vi "CLD1010 Example.vi"() -> ()   [LabVIEW 2023]
panel:
  in  "Resource Name":refnum<visa-resource-name>="USB0::0x1313::0x804F::M00413716::INSTR"
  out "Temperature High Limit":dbl caption="Setpoint High Limit"
  out "Temperature  Low Limit":dbl caption="Setpoint Low Limit"
  in  "Laser Diode Current Setpoint [A] (0.0)":dbl caption="Laser Diode Current Setpoint (0.0)"
  out "Measured Temperature":dbl caption="Temperature"
  in  "Temperature Setpoint [°C] (25.0)":dbl=25.0 caption="Temperature Setpoint (25.0)"
  # "CLD1010 Example"
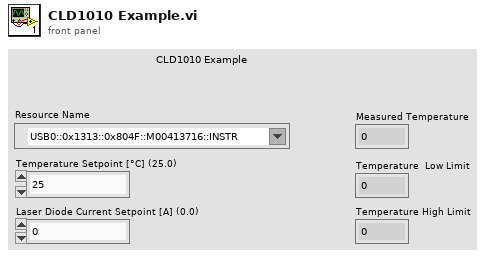
[diagram p1: front panel]
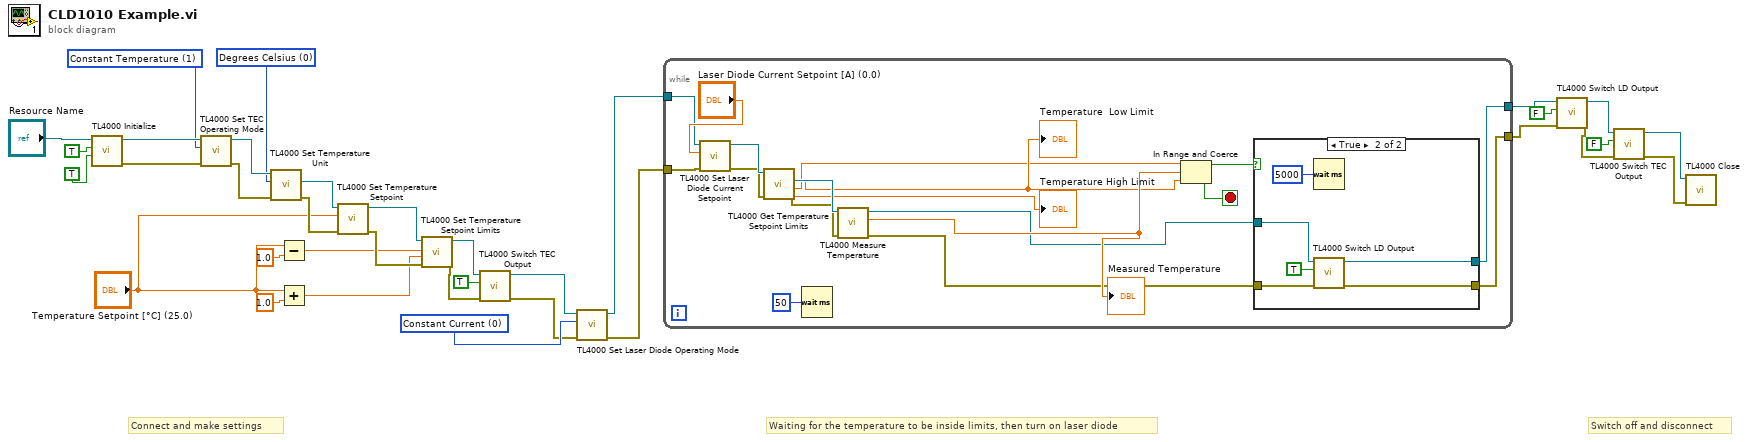
[diagram p0: block diagram]
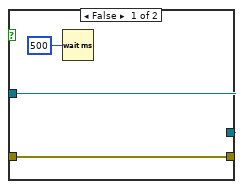
[diagram p2: hidden frame]
diagram:
  w21 = i16 1 items=["Constant Temperature"=1, "Current Source"=0] ("TEC Operating Mode (Constant Temperature)")
  w22 = i16 0 items=["Degrees Celsius", "Kelvin", "Degrees Fahrenheit"] ("Temperature Unit (Degrees Celsius)")
  w27 = i16 0 items=["Constant Current", "Constant Power"] ("Laser Diode Operating Mode (Constant Current)")
  # "Switch off and disconnect"
  # "Waiting for the temperature to be inside limits, then turn on laser diode"
  # "Connect and make settings"
  n1 = call <instrlib>:"TL4000 Initialize.vi"("Reset Device (Reset Device)"=TRUE, "ID Query (Do Query)"=TRUE, "resource name"="Resource Name") -> ("error out"=w1:errorcluster, "instrument handle out"=w31:refnum<visa-resource-name>)  [unwired: 7 in]
  n2 = call <instrlib>:"TL4000 Set TEC Operating Mode.vi"("error in (no error)"=w1, "TEC Operating Mode (Constant Temperature)"=w21, "instrument handle"=w31) -> ("error out"=w24:errorcluster, "instrument handle out"=w26:refnum<visa-resource-name>)  [unwired: 7 in]
  n3 = call <instrlib>:"TL4000 Set Temperature Unit.vi"("error in (no error)"=w24, "Temperature Unit (Degrees Celsius)"=w22, "instrument handle"=w26) -> ("error out"=w23:errorcluster, "instrument handle out"=w25:refnum<visa-resource-name>)  [unwired: 7 in]
  n4 = Subtract(x="Temperature Setpoint [°C] (25.0)", y=1.0) -> (x-y=w2:dbl)
  n5 = Add(x="Temperature Setpoint [°C] (25.0)", y=1.0) -> (x+y=w5:dbl)
  n6 = call <instrlib>:"TL4000 Set Temperature Setpoint.vi"("error in (no error)"=w23, "Temperature Setpoint (25.0)"="Temperature Setpoint [°C] (25.0)", "instrument handle"=w25) -> ("error out"=w8:errorcluster, "instrument handle out"=w10:refnum<visa-resource-name>)  [unwired: 7 in]
  n7 = call "TL4000 Set Temperature Setpoint Limits.vi"("error in (no error)"=w8, "Setpoint High Limit (50.0)"=w5, "Setpoint Low Limit (0.0)"=w2, "instrument handle"=w10) -> ("error out"=w7:errorcluster, "instrument handle out"=w9:refnum<visa-resource-name>)  [unwired: 6 in]
  n8 = call <instrlib>:"TL4000 Switch TEC Output.vi"("error in (no error)"=w7, "TEC Output (Off)"=TRUE, "instrument handle"=w9) -> ("error out"=w19:errorcluster, "instrument handle out"=w20:refnum<visa-resource-name>)  [unwired: 7 in]
  n9 = call <instrlib>:"TL4000 Set Laser Diode Operating Mode.vi"("error in (no error)"=w19, "Laser Diode Operating Mode (Constant Current)"=w27, "instrument handle"=w20) -> ("error out"=w29:errorcluster, "instrument handle out"=w28:refnum<visa-resource-name>)  [unwired: 7 in]
  n10 = while {
    tunnel: w29 -> [w44]
    tunnel: w28 -> [w45]
    tunnel: [w42] -> w15
    tunnel: [w41] -> w14
    stop <- w43 stop-if-true
    n11 = call <instrlib>:"TL4000 Set Laser Diode Current Setpoint.vi"("error in (no error)"=w44, "Laser Diode Current Setpoint (0.0)"="Laser Diode Current Setpoint [A] (0.0)", "instrument handle"=w45) -> ("error out"=w39:errorcluster, "instrument handle out"=w40:refnum<visa-resource-name>)  [unwired: 7 in]
    n12 = call "TL4000 Get Temperature Setpoint Limits.vi"("error in (no error)"=w39, "instrument handle"=w40) -> ("error out"=w37:errorcluster, "Setpoint High Limit"=w35:dbl, "Setpoint Low Limit"=w36:dbl, "instrument handle out"=w38:refnum<visa-resource-name>)  [unwired: 6 in]
    "Temperature  Low Limit" <- w36
    "Temperature High Limit" <- w35
    n13 = Wait (ms)(milliseconds to wait=u32 50) -> ()  [unwired: 1 out]
    n14 = call <instrlib>:"TL4000 Measure Temperature.vi"("error in (no error)"=w37, "instrument handle"=w38) -> ("error out"=w47:errorcluster, "Temperature"=w49:dbl, "instrument handle out"=w48:refnum<visa-resource-name>)  [unwired: 7 in]
    "Measured Temperature" <- w49
    n15 = In Range and Coerce(upper limit=w35, x=w49, lower limit=w36) -> (In Range?=w43:bool)  [unwired: 1 out]
    n16 = case shown="True" w43 {
      tunnel: w48 -> [w53 w58]
      tunnel: w47 -> [w52 w57]
      tunnel: [w53 w54] -> w41
      tunnel: [w52 w55] -> w42
      frame False {
        n17 = Wait (ms)(milliseconds to wait=u32 500) -> ()  [unwired: 1 out]
      }
      frame True {
        n18 = Wait (ms)(milliseconds to wait=u32 5000) -> ()  [unwired: 1 out]
        n19 = call <instrlib>:"TL4000 Switch LD Output.vi"("error in (no error)"=w57, "LD Output (Off)"=TRUE, "instrument handle"=w58) -> ("error out"=w55:errorcluster, "instrument handle out"=w54:refnum<visa-resource-name>)  [unwired: 7 in]
      }
    }
  }
  n20 = call <instrlib>:"TL4000 Switch LD Output.vi"("error in (no error)"=w15, "LD Output (Off)"=FALSE, "instrument handle"=w14) -> ("error out"=w13:errorcluster, "instrument handle out"=w12:refnum<visa-resource-name>)  [unwired: 7 in]
  n21 = call <instrlib>:"TL4000 Switch TEC Output.vi"("error in (no error)"=w13, "TEC Output (Off)"=FALSE, "instrument handle"=w12) -> ("error out"=w18:errorcluster, "instrument handle out"=w17:refnum<visa-resource-name>)  [unwired: 7 in]
  n22 = call <instrlib>:"TL4000 Close.vi"("error in (no error)"=w18, "instrument handle"=w17) -> ()  [unwired: 9 in, 1 out]
